vi "SaveQueueCluster.vi"() -> ()   [LabVIEW 2017]
uses:
  SaveQueueCluster.ctl
  SaveMessage.ctl
panel:
  in  "SaveQueueCluster":T1
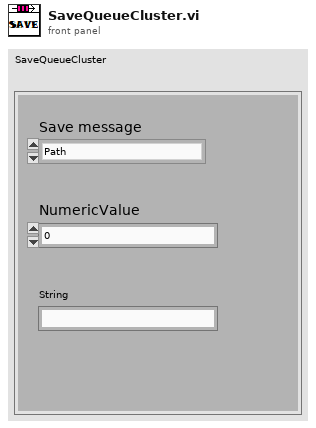
[diagram p1: front panel]
types:
  T1 = typedef "SaveQueueCluster.ctl" = cluster{"Save message":T2, "NumericValue":dbl, "String":string}
  T2 = typedef "SaveMessage.ctl" = enum16{"Path", "StartSaving", "StopSaving", "Ch1Value", "Ch2Value", "Ch3Value"}
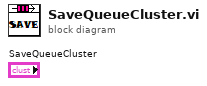
[diagram p0: block diagram]
diagram:
